vi "getITaskClassTemplatePath.vi"() -> (0 "ITaskClassPath":path)   [LabVIEW 2023]
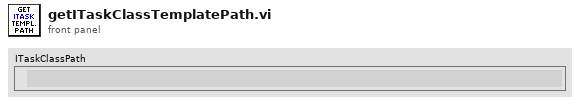
[diagram p1: front panel]
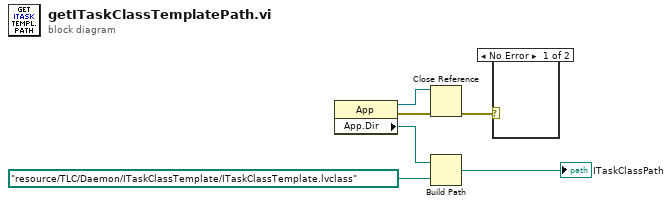
[diagram p0: block diagram]
diagram:
  n1 = property class="App"() -> (reference out=w4:refnum<vi>, error out=w5:errorcluster, "App.Dir"=w3:path)  [unwired: 2 in]
  n2 = Close Reference(reference=w4, error in (no error)=w5) -> (error out=w6:errorcluster)
  n3 = Build Path(base path=w3, name or relative path=path "resource/TLC/Daemon/ITaskClassTemplate/ITaskClassTemplate.lvclass") -> (appended path=→"ITaskClassPath":path)
  n4 = case shown="No Error" w6 {
    frame No Error {
    }
    frame Error {
    }
  }
